vi "find_zip_file_for_xml.vi"(8 "error in (no error)":errorcluster, 10 "xml file in":path) -> (0 "error out":errorcluster, 1 "file or folder exists?":bool, 2 "new zip file out":path)   [LabVIEW 2010, in "ErrorController.lvclass"]
uses:
  ErrorController.lvclass
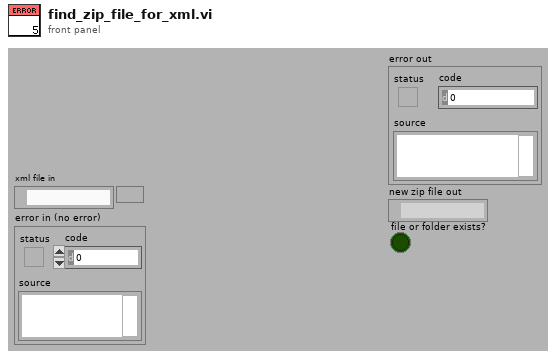
[diagram p1: front panel]
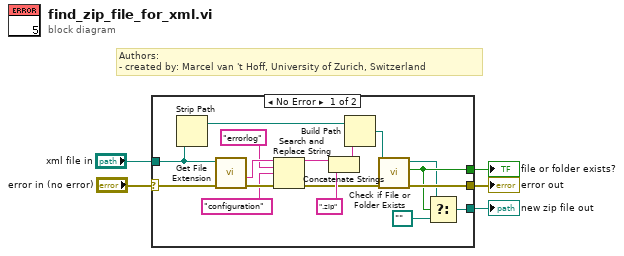
[diagram p0: block diagram]
diagram:
  # "Authors: \n- created by: Marcel van 't Hoff, University of Zurich, Switzerland"
  n1 = case shown="No Error" "error in (no error)" {
    selector: "error in (no error)" -> [w22 w23]
    tunnel: "xml file in" -> [w17 _]
    tunnel: [w6 _] -> w2
    tunnel: [w9 _] -> w1
    tunnel: [w10 w23] -> w3
    frame No Error {
      n2 = Strip Path(path=w17) -> (stripped path=w16:path)  [unwired: 1 out]
      n3 = call <vilib>:"Get File Extension.vi"("error in (no error)"=w22, "file"=w17) -> ("error out"=w20:errorcluster, "filename without extension"=w21:string)  [unwired: 6 in, 2 out]
      n4 = Search and Replace String(input string=w21, search string="errorlog", replace string="configuration" ("replace string (\"\")"), error in=w20) -> (result string=w15:string, error out=w12:errorcluster)  [unwired: 4 in, 2 out]
      n5 = Concatenate Strings(w15, ".zip" ("string")) -> (w13:string)
      n6 = Build Path(base path=w16, name or relative path=w13) -> (appended path=w11:path)
      n7 = call <vilib>:"Check if File or Folder Exists.vi"("error in (no error)"=w12, "path"=w11) -> ("error out"=w10:errorcluster, "file or folder exists?"=w9:bool, "dup path"=w7:path)  [unwired: 7 in]
      n8 = Select(t=w7, s=w9, f=path "") -> (s? t:f=w6:path)
    }
    frame Error {
    }
  }
  "error out" <- w3
  "new zip file out" <- w2
  "file or folder exists?" <- w1
